vi "deferUpdates.vi"(7 "DVR":T1, 10 "defer?":bool) -> ()   [LabVIEW 2020]
uses:
  _controls/data.ref.ctl
  _controls/state.ctl
  _controls/flip.ctl
  _controls/data.vars.ctl
  _controls/data.ctl
  <vilib>/vision/Image Controls.llb/IMAQ Image.ctl
  camera/camera.lvclass
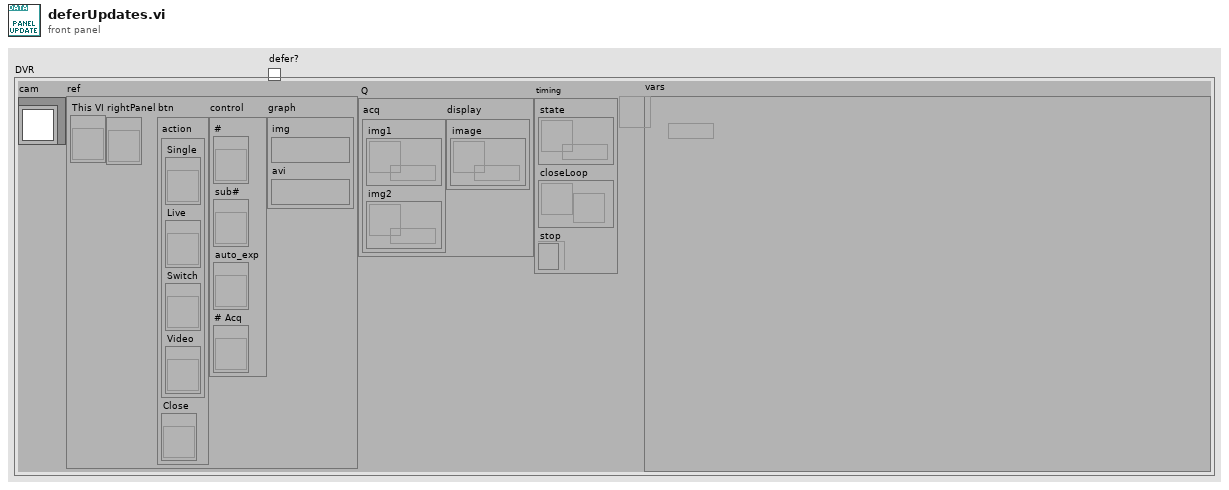
[diagram p1: front panel]
types:
  T1 = typedef "data.ctl" = cluster{"cam":refnum<class "camera.lvclass">, "ref":T2, "Q":cluster{"acq":cluster{"img1":refnum<queue>, "img2":refnum<queue>}, "display":cluster{"image":refnum<queue>}}, "timing":cluster{"state":refnum<queue>, "closeLoop":refnum<notifier>, "stop":refnum<k4>}, "vars":refnum<data-value>}
  T2 = typedef "data.ref.ctl" = cluster{"This VI":refnum<vi>, "rightPanel":refnum<vi>, "btn":cluster{"action":cluster{"Single":refnum<vi>, "Live":refnum<vi>, "Switch":refnum<vi>, "Video":refnum<vi>}, "Close":refnum<vi>}, "control":cluster{"#":refnum<vi>, "sub#":refnum<vi>, "auto_exp":refnum<vi>, "# Acq":refnum<vi>}, "graph":cluster{"img":T3, "avi":T3}}
  T3 = typedef "IMAQ Image.ctl" = refnum<image>
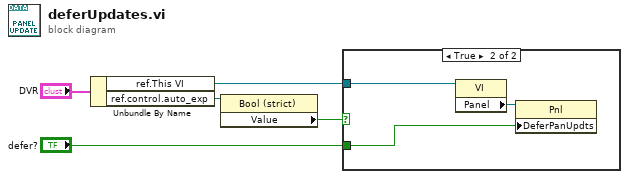
[diagram p0: block diagram]
diagram:
  n1 = Unbundle By Name("DVR") -> ("ref.This VI"=w3:refnum<vi>, "ref.control.auto_exp"=w2:refnum<vi>)
  n2 = property class="Bool (strict)"(reference=w2) -> ("Value"=w1:bool)  [unwired: 1 in, 2 out]
  n3 = case shown="True" w1 {
    tunnel: "defer?" -> [_ w8]
    tunnel: w3 -> [_ w6]
    frame False {
    }
    frame True {
      n4 = property class="VI"(reference=w6) -> ("Panel"=w7:refnum<vi>)  [unwired: 1 in, 2 out]
      n5 = property class="Pnl"(reference=w7, "DeferPanUpdts"=w8) -> ()  [unwired: 1 in, 2 out]
    }
  }
